vi "RintSweep.vi"(0 "Action":enum16{"Reset", "Measure"}(ring), 5 "MasterVoltage Supply in":refnum<class "SupplyControl.lvclass">, 7 "VoltmeterControl in":refnum<class "MultimeterControl.lvclass">, 9 "No. of readouts":i32, 11 "Bias [V]":dbl, 12 "Simulated data?":bool) -> (2 "Sweep":i32[](array[numeric])=[0, -1, -2, -3, -4, -5, -4, -3, -2, -1, 0, 1, 2, 3, 4, 5, 4, 3, 2, 1, 0], 3 "Igraph":cluster{i32[], dbl[]}[](graph), 4 "Applied Current [nA]":dbl[][][](array[numeric]), 6 "Induced Voltage [V]":dbl[][][](array[numeric]), 8 "Voltages OUT":dbl[](array[numeric]), 10 "Compliance exceeded?":bool, 14 "ViGraph":cluster{i32[], dbl[]}[](graph), 15 "Error Out":errorcluster)   [LabVIEW 2013]
uses:
  InstrControl/SupplyControl/SupplyControl.lvclass
  InstrControl/MultimeterControl/MultimeterControl.lvclass
panel:
  in  "Error In":errorcluster
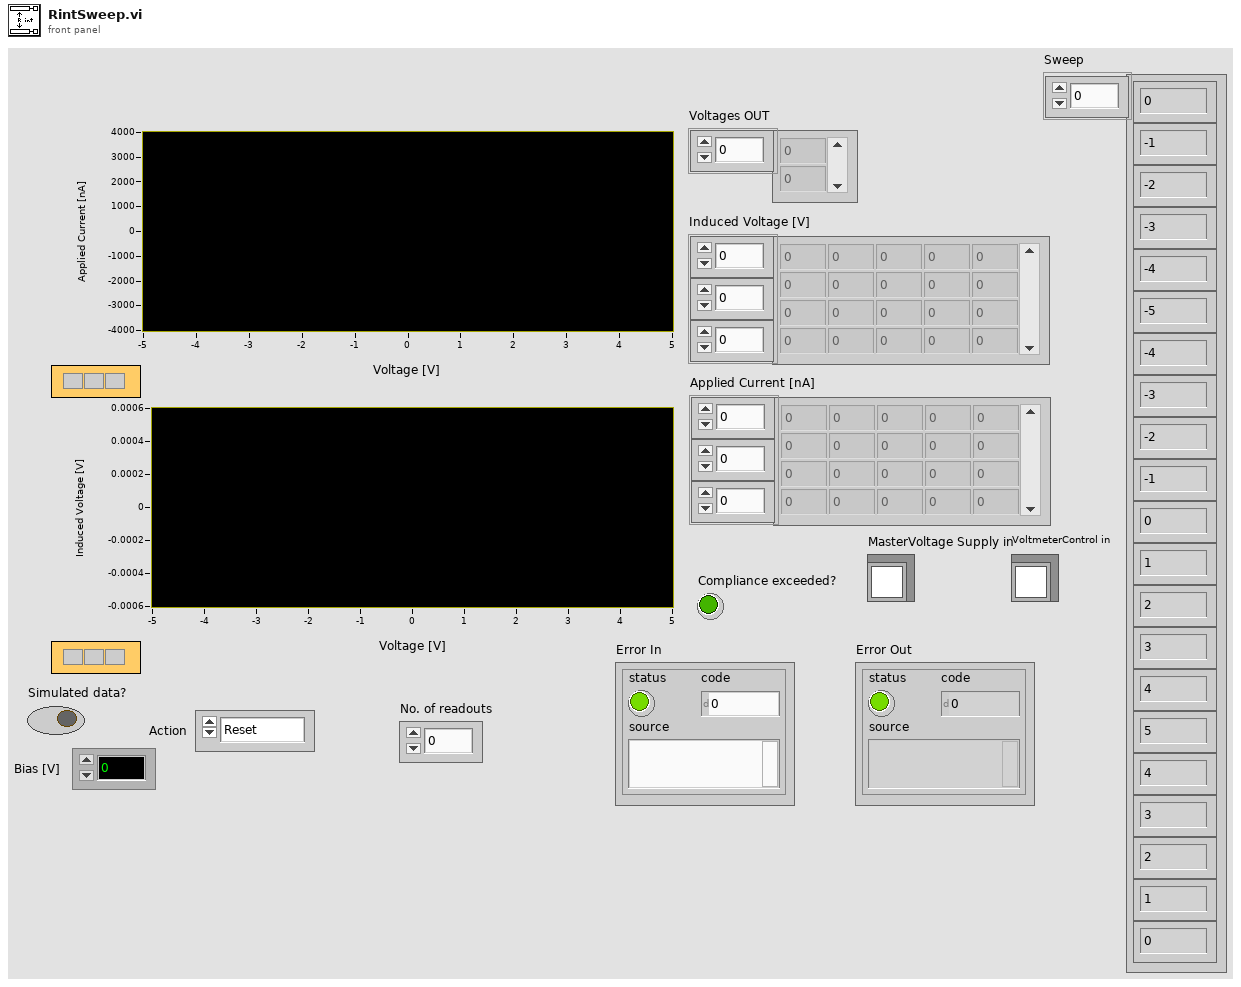
[diagram p1: front panel]
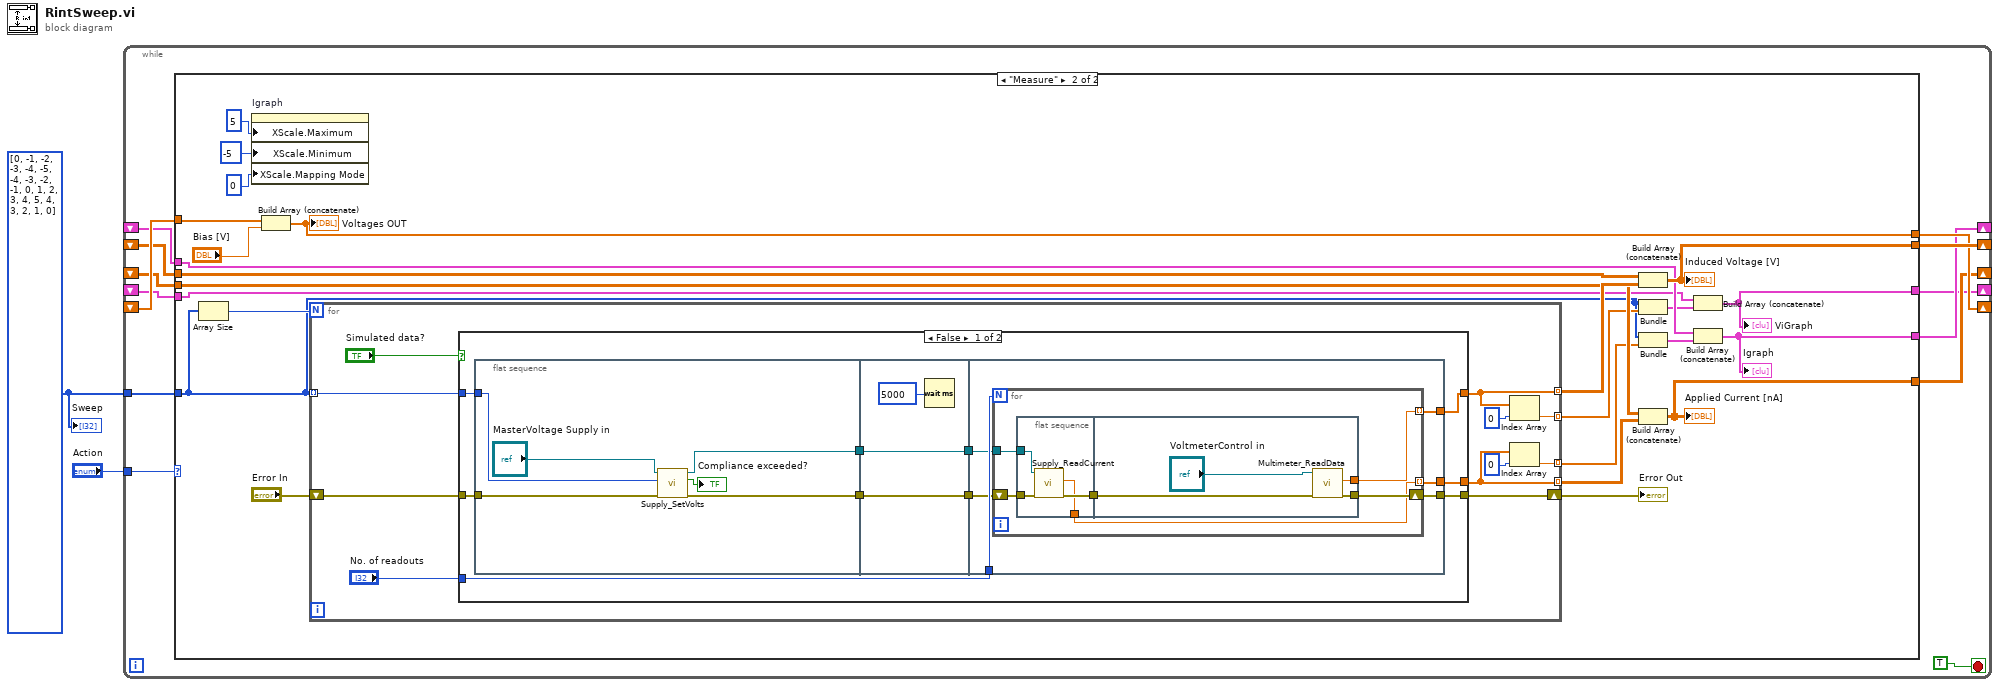
[diagram p0: block diagram]
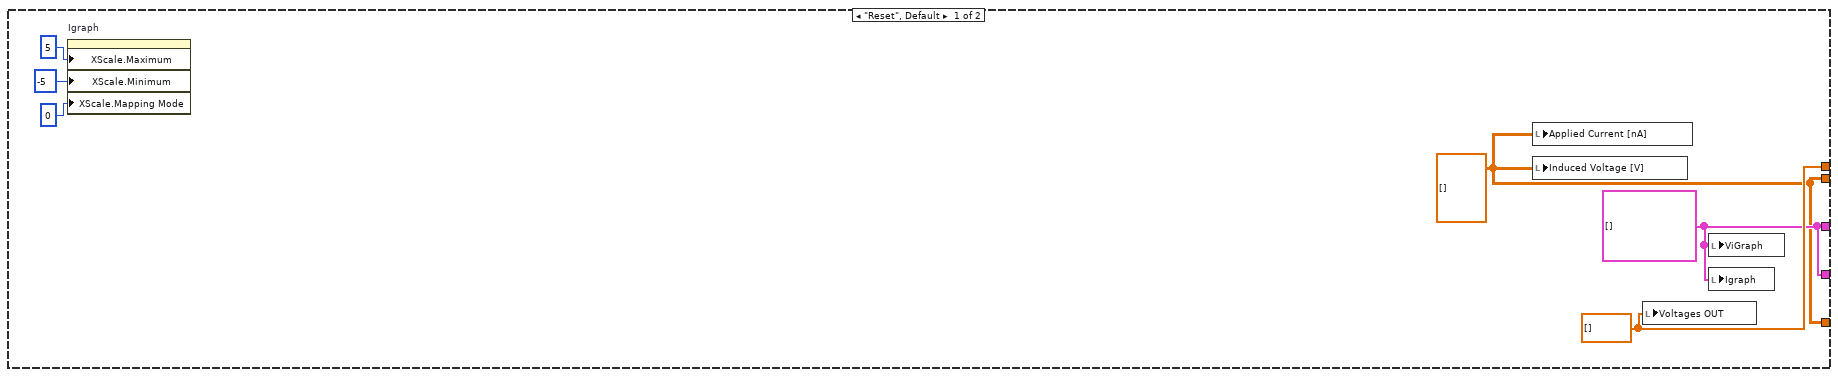
[diagram p2: hidden frame]
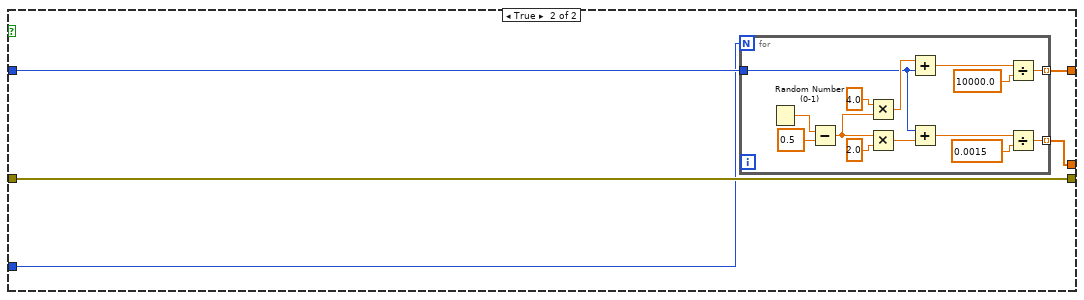
[diagram p3: hidden frame]
diagram:
  w1 = i32[] [0, -1, -2, -3, -4, -5, -4, -3, -2, -1, 0, 1, 2, 3, 4, 5, 4, 3, 2, 1, 0]
  n1 = while {
    tunnel: w1 -> [w15]
    tunnel: "Action" -> [w13]
    shift-right: [w12] -> _
    shift-left: _ -> [w8]
    shift-right: [w11] -> _
    shift-left: _ -> [w9]
    shift-right: [w10] -> _
    shift-left: _ -> [w7]
    shift-right: [w6] -> _
    shift-left: _ -> [w5]
    shift-right: [w4] -> _
    shift-left: _ -> [w3]
    stop <- TRUE stop-if-true
    n2 = case shown="\"Measure\"" w13 {
      tunnel: w15 -> [_ w23]
      tunnel: [w16 w37] -> w12
      tunnel: [w18 w39] -> w11
      tunnel: [w17 w36] -> w10
      tunnel: w9 -> [_ w40]
      tunnel: w8 -> [_ w38]
      tunnel: w7 -> [_ w35]
      tunnel: [w16 w28] -> w6
      tunnel: w5 -> [_ w30]
      tunnel: [w17 w26] -> w4
      tunnel: w3 -> [_ w25]
      frame "Reset", Default {
        w16 = dbl[][][] []
        w17 = cluster{i32[], dbl[]}[] []
        w18 = dbl[] []
        n3 = property on="Igraph" class="XYGraph (strict)"("XScale.Maximum"=5, "XScale.Minimum"=-5, "XScale.Mapping Mode"=0) -> ()  [unwired: 2 in, 2 out]
        n4 = local write "Applied Current [nA]"(w16) -> ()
        n5 = local write "Induced Voltage [V]"(w16) -> ()
        n6 = local write "Voltages OUT"(w18) -> ()
        n7 = local write "ViGraph"(w17) -> ()
        n8 = local write "Igraph"(w17) -> ()
      }
      frame "Measure" {
        n9 = Array Size(array=w23) -> (size(s)=w45:i32)
        n10 = property on="Igraph" class="XYGraph (strict)"("XScale.Maximum"=5, "XScale.Minimum"=-5, "XScale.Mapping Mode"=0) -> ()  [unwired: 2 in, 2 out]
        n11 = Build Array (concatenate)(w40, "Bias [V]") -> (w39:dbl[])
        "Voltages OUT" <- w39
        n12 = for {
          N: w45 -> [_]
          tunnel: w23 -> [w55] mode=indexing
          tunnel: [w47] -> w34 mode=indexing
          shift-right: [w53] -> w31
          shift-left: "Error In" -> [w54]
          tunnel: [w50] -> w22 mode=indexing
          tunnel: [w49] -> w29 mode=indexing
          tunnel: [w46] -> w24 mode=indexing
          n13 = case shown="False" "Simulated data?" {
            tunnel: w55 -> [w62 w100]
            tunnel: [w66 w96] -> w47
            tunnel: w54 -> [w63 w99]
            tunnel: [w65 w99] -> w53
            tunnel: "No. of readouts" -> [w64 w98]
            tunnel: [w61 w97] -> w49
            frame False {
              n14 = flat-sequence {
                tunnel: w63 -> [w71]
                tunnel: w62 -> [w72]
                tunnel: [w70] -> w60
                tunnel: [w69] -> w57
                tunnel: w60 -> [w75]
                tunnel: [w75] -> w59
                tunnel: [w73] -> w58
                tunnel: w57 -> [w73]
                tunnel: [w81] -> w66
                tunnel: [w80] -> w65
                tunnel: w64 -> [w79]
                tunnel: w59 -> [w78]
                tunnel: [w77] -> w61
                tunnel: w58 -> [w76]
                frame #0 {
                  n15 = call-dynamic "Supply_SetVolts.vi"("error in (no error)"=w71, "Volts IN [V]"=w72, "SupplyControl in"="MasterVoltage Supply in") -> ("error out"=w70:errorcluster, "Compliance exceeded?"=→"Compliance exceeded?":bool, "SupplyControl out"=w69:refnum<class "SupplyControl.lvclass">)  [unwired: 6 in]
                }
                frame #1 {
                  n16 = Wait (ms)(milliseconds to wait=5000) -> ()  [unwired: 1 out]
                }
                frame #2 {
                  n17 = for {
                    N: w79 -> [_]
                    tunnel: [w87] -> w81 mode=indexing
                    shift-right: [w85] -> w80
                    shift-left: w78 -> [w86]
                    tunnel: [w83] -> w77 mode=indexing
                    tunnel: w76 -> [w82]
                    n18 = flat-sequence {
                      tunnel: w86 -> [w91]
                      tunnel: [w90] -> w84
                      tunnel: [w89] -> w83
                      tunnel: w82 -> [w88]
                      tunnel: [w92] -> w87
                      tunnel: [w93] -> w85
                      tunnel: w84 -> [w95]
                      frame #0 {
                        n19 = call-dynamic "Supply_ReadCurrent.vi"("error in (no error)"=w91, "SupplyControl in"=w88) -> ("error out"=w90:errorcluster, "Current in nA"=w89:dbl)  [unwired: 7 in, 1 out]
                      }
                      frame #1 {
                        n20 = call-dynamic "Multimeter_ReadData.vi"("error in (no error)"=w95, "MultimeterControl in"="VoltmeterControl in") -> ("error out"=w93:errorcluster, "Voltage in V"=w92:dbl)  [unwired: 7 in, 1 out]
                      }
                    }
                  }
                }
              }
            }
            frame True {
              n21 = for {
                N: w98 -> [_]
                tunnel: w100 -> [w108]
                tunnel: [w101] -> w97 mode=indexing
                tunnel: [w104] -> w96 mode=indexing
                n22 = Random Number (0-1)() -> (number: 0 to 1=w114:dbl)
                n23 = Subtract(x=w114, y=0.5) -> (x-y=w106:dbl)
                n24 = Multiply(x=4.0, y=w106) -> (x*y=w110:dbl)
                n25 = Multiply(x=w106, y=2.0) -> (x*y=w105:dbl)
                n26 = Add(x=w110, y=w108) -> (x+y=w109:dbl)
                n27 = Add(x=w108, y=w105) -> (x+y=w102:dbl)
                n28 = Divide(x=w109, y=10000.0) -> (x/y=w104:dbl)
                n29 = Divide(x=w102, y=0.0015) -> (x/y=w101:dbl)
              }
            }
          }
          n30 = Index Array(array=w47, index=0) -> (element=w46:dbl)
          n31 = Index Array(array=w49, index=0) -> (element=w50:dbl)
        }
        "Error Out" <- w31
        n32 = Build Array (concatenate)(w38, w34) -> (w37:dbl[][][])
        "Induced Voltage [V]" <- w37
        n33 = Bundle(w23, w24) -> (w27:cluster{i32[], dbl[]})  [unwired: 1 in]
        n34 = Bundle(w23, w22) -> (w33:cluster{i32[], dbl[]})  [unwired: 1 in]
        n35 = Build Array (concatenate)(w30, w29) -> (w28:dbl[][][])
        "Applied Current [nA]" <- w28
        n36 = Build Array (concatenate)(w25, w27) -> (w26:cluster{i32[], dbl[]}[])
        "ViGraph" <- w26
        n37 = Build Array (concatenate)(w35, w33) -> (w36:cluster{i32[], dbl[]}[])
        "Igraph" <- w36
      }
    }
  }
  "Sweep" <- w1
